vi "Test EfficientNet_B4.vi"() -> ()   [LabVIEW 2017]
doc: "Created IvanLis by LabVIEW Portal\nProfile: http://labviewportal.org/memberlist.php?mode=viewprofile&u=987\neMail: IvanLisanov@gMail.com\nTelegram: https://t.me/IvanLis"
uses:
  libonnx_wrapper/libonnx_wrapper.lvlib
  process_YOLOv8/process_YOLOv8.lvlib
  process_Angle/process_Angle.lvlib
  process_EfficientNet_B4/process_EfficientNet_B4.lvlib
panel:
  out "Result":T1(array[cluster])
  out "Spin Image":picture[](array[picture])
  out "2D Picture":picture
  in  "BMP file path":path=path "/home/ivan/LabVIEWData/ONNX/LabVIEW-ONNX_Runtime/image_for_test/2005mmd_b2_1r_2005mmd_b2_var33.jpg"
  out "error out":errorcluster
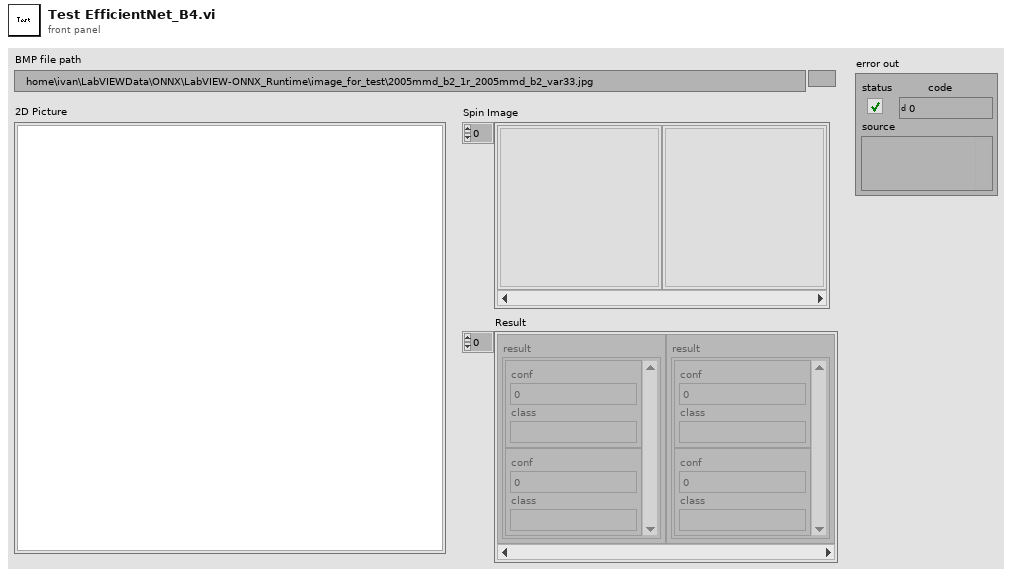
[diagram p1: front panel]
types:
  T1 = cluster{"result":cluster{"conf":sgl, "class":string}[]}[]
  T2 = typedef "imagedata.ctl" = cluster{"image type":i32, "image depth":i32, "image":u8[], "mask":u8[], "colors":u32[], "Rectangle":cluster{"left":i16, "top":i16, "right":i16, "bottom":i16}}
  T3 = typedef "libonnx_wrapper.lvlib/Introspection.ctl" = cluster{"Count":i32, "Shapes":T4[]}
  T4 = typedef "libonnx_wrapper.lvlib/IO.ctl" = cluster{"Name":string, "DimCount":i32, "Type Index":i32, "Type Name":string, "Dims":i64[]}
  T5 = typedef "process_YOLOv8.lvlib/Circle.ctl" = cluster{"x":sgl, "y":sgl, "r":sgl}
  T6 = cluster{"result":cluster{"conf":sgl, "class":string}[]}
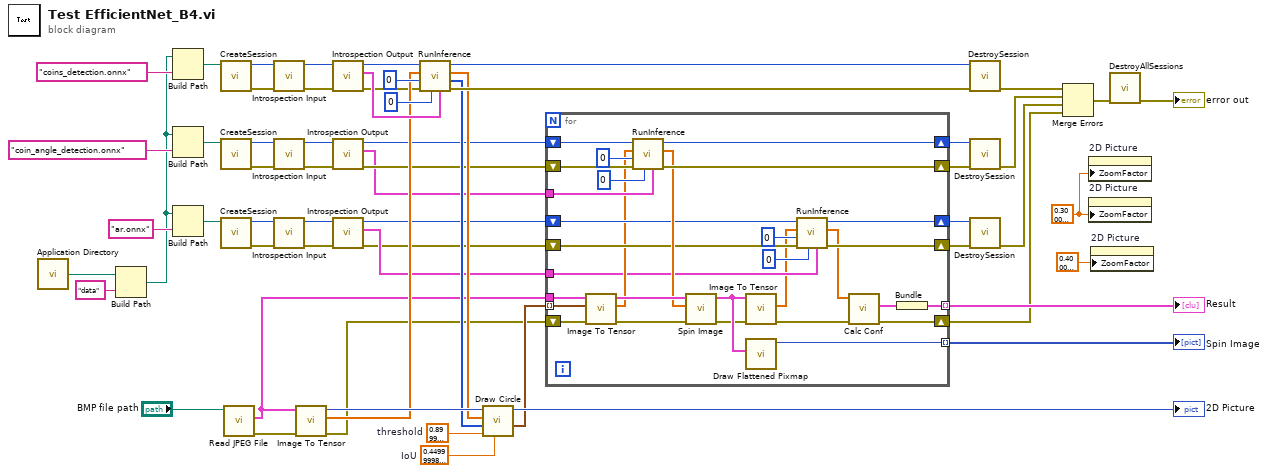
[diagram p0: block diagram]
diagram:
  w30 = sgl 0.3 ("Zoom Factor")
  w40 = sgl 0.45  # IoU
  w41 = sgl 0.9  # threshold
  n1 = call <vilib>:"Application Directory.vi"() -> ("Application Directory"=w25:path)
  n2 = Build Path(base path=w25, name or relative path="data") -> (appended path=w7:path)
  n3 = Build Path(base path=w7, name or relative path="coins_detection.onnx") -> (appended path=w23:path)
  n4 = Build Path(base path=w7, name or relative path="coin_angle_detection.onnx") -> (appended path=w21:path)
  n5 = Build Path(base path=w7, name or relative path="ar.onnx") -> (appended path=w16:path)
  n6 = call "CreateSession.vi"("ONNX model path"=w23) -> ("error out"=w51:errorcluster, "session id out"=w52:i32)  [unwired: 9 in]
  n7 = call "CreateSession.vi"("ONNX model path"=w21) -> ("error out"=w35:errorcluster, "session id out"=w34:i32)  [unwired: 9 in]
  n8 = call "CreateSession.vi"("ONNX model path"=w16) -> ("error out"=w12:errorcluster, "session id out"=w13:i32)  [unwired: 9 in]
  n9 = call <vilib>:"Read JPEG File.vi"("path to JPEG file"="BMP file path") -> ("error out"=w53:errorcluster, "image data"=w39:T2)  [unwired: 8 in, 1 out]
  n10 = call "Introspection Input.vi"("error in (no error)"=w51, "session id in"=w52) -> ("error out"=w58:errorcluster, "session id out"=w59:i32)  [unwired: 7 in, 1 out]
  n11 = call "Introspection Input.vi"("error in (no error)"=w35, "session id in"=w34) -> ("error out"=w33:errorcluster, "session id out"=w32:i32)  [unwired: 7 in, 1 out]
  n12 = call "Introspection Input.vi"("error in (no error)"=w12, "session id in"=w13) -> ("error out"=w14:errorcluster, "session id out"=w15:i32)  [unwired: 7 in, 1 out]
  n13 = call "Image To Tensor.vi"("error in (no error)"=w53, "image data"=w39) -> ("error out"=w3:errorcluster, "Data"=w44:sgl[], "image"=w48:picture)  [unwired: 7 in]
  n14 = call "Introspection Output.vi"("error in (no error)"=w58, "session id in"=w59) -> ("error out"=w26:errorcluster, "Introspection Output"=w46:T3, "session id out"=w27:i32)  [unwired: 7 in]
  n15 = call "Introspection Output.vi"("error in (no error)"=w33, "session id in"=w32) -> ("error out"=w18:errorcluster, "Introspection Output"=w1:T3, "session id out"=w19:i32)  [unwired: 7 in]
  n16 = call "Introspection Output.vi"("error in (no error)"=w14, "session id in"=w15) -> ("error out"=w5:errorcluster, "Introspection Output"=w8:T3, "session id out"=w6:i32)  [unwired: 7 in]
  n17 = call "RunInference.vi"("Introspection Output"=w46, "outputIndex"=0, "error in (no error)"=w26, "inputIndex"=0, "inputBuffer"=w44, "session id in"=w27) -> ("error out"=w50:errorcluster, "Dims"=w43:i64[], "outputBuffer"=w42:sgl[], "session id out"=w49:i32)  [unwired: 2 in]
  n18 = call "Draw Circle.vi"("IoU"=w40, "threshold"=w41, "dim"=w43, "data"=w42, "image in"=w48) -> ("Circles"=w29:T5[], "image out"=→"2D Picture":picture)  [unwired: 4 in, 1 out]
  n19 = for {
    tunnel: w39 -> [w90]
    tunnel: w1 -> [w83]
    shift-right: [w87] -> w36
    shift-left: w18 -> [w85]
    shift-right: [w88] -> w37
    shift-left: w19 -> [w84]
    tunnel: w29 -> [w79] mode=indexing
    tunnel: [w78] -> w28 mode=indexing
    shift-right: [w76] -> w10
    shift-left: w6 -> [w77]
    shift-right: [w74] -> w9
    shift-left: w5 -> [w75]
    tunnel: w8 -> [w70]
    tunnel: [w63] -> w4 mode=indexing
    shift-right: [w61] -> w2
    shift-left: w3 -> [w62]
    n20 = call "Image To Tensor.vi"("error in (no error)"=w62, "Circle"=w79, "image data IN"=w90) -> ("error out"=w80:errorcluster, "Data"=w71:sgl[], "image data OUT"=w82:T2)  [unwired: 5 in, 1 out]
    n21 = call "RunInference.vi"("Introspection Output"=w83, "outputIndex"=0, "error in (no error)"=w85, "inputIndex"=0, "inputBuffer"=w71, "session id in"=w84) -> ("error out"=w87:errorcluster, "outputBuffer"=w81:sgl[], "session id out"=w88:i32)  [unwired: 2 in, 1 out]
    n22 = call "Spin Image.vi"("error in (no error)"=w80, "data"=w81, "image data IN"=w82) -> ("error out"=w68:errorcluster, "image data OUT"=w69:T2)  [unwired: 6 in, 1 out]
    n23 = call "Image To Tensor.vi"("error in (no error)"=w68, "image data IN"=w69) -> ("error out"=w65:errorcluster, "Data"=w67:sgl[])  [unwired: 8 in]
    n24 = call <vilib>:"Draw Flattened Pixmap.vi"("image data"=w69) -> ("new picture"=w78:picture)  [unwired: 8 in]
    n25 = call "RunInference.vi"("Introspection Output"=w70, "outputIndex"=0, "error in (no error)"=w75, "inputIndex"=0, "inputBuffer"=w67, "session id in"=w77) -> ("error out"=w74:errorcluster, "outputBuffer"=w66:sgl[], "session id out"=w76:i32)  [unwired: 2 in, 1 out]
    n26 = call "Calc Conf.vi"("error in (no error)"=w65, "data"=w66) -> ("error out"=w61:errorcluster, "result"=w64:cluster{"conf":sgl, "class":string}[])  [unwired: 7 in, 1 out]
    n27 = Bundle("result"=w64) -> (w63:T6)  [unwired: 1 in]
  }
  "Spin Image" <- w28
  "Result" <- w4
  n28 = call "DestroySession.vi"("error in (no error)"=w50, "session id in"=w49) -> ("error out"=w60:errorcluster)  [unwired: 8 in, 1 out]
  n29 = call "DestroySession.vi"("error in (no error)"=w36, "session id in"=w37) -> ("error out"=w31:errorcluster)  [unwired: 8 in, 1 out]
  n30 = call "DestroySession.vi"("error in (no error)"=w9, "session id in"=w10) -> ("error out"=w11:errorcluster)  [unwired: 8 in, 1 out]
  n31 = Merge Errors(w60, w31, w11, w2) -> (w38:errorcluster)
  n32 = property on="2D Picture" class="Pict"("ZoomFactor"=w30) -> ()  [unwired: 2 in, 2 out]
  n33 = property on="2D Picture" class="Pict"("ZoomFactor"=w30) -> ()  [unwired: 2 in, 2 out]
  n34 = property on="2D Picture" class="Pict"("ZoomFactor"=sgl 0.4 ("Zoom Factor")) -> ()  [unwired: 2 in, 2 out]
  n35 = call "DestroyAllSessions.vi"("error in (no error)"=w38) -> ("error out"=→"error out":errorcluster)  [unwired: 10 in]
